vi "Load Firmware Data.vi"(8 "Error In":errorcluster, 9 "Firmware Index":i32, 10 "Device Index":i32, 11 "Family Index":i32) -> (0 "Error Out":errorcluster, 2 "Firmware Interface":T1, 3 "Firmware Description":string)   [LabVIEW 2011, in "LVH-LINX.lvlib"]
doc: "Load specified firmware readme."
uses:
  LVH-LINX.lvlib
  Device/Type Defs/Firmware Interface.ctl
  Type Defs/All Firmware Data FGV States.ctl
panel:
  in  "Device Family":u16(ring) items=["National Instruments", "Digilent", "Arduino"]
  in  "Device Type":u16(ring) items=["chipKIT Uno32", "chipKIT uC32", "chipKIT Max32", "chipKIT DP32"]
  in  "Firmware Version":u16(ring) items=["LINX -  Serial / USB", "LINX -  Serial / USB [Debug] "]
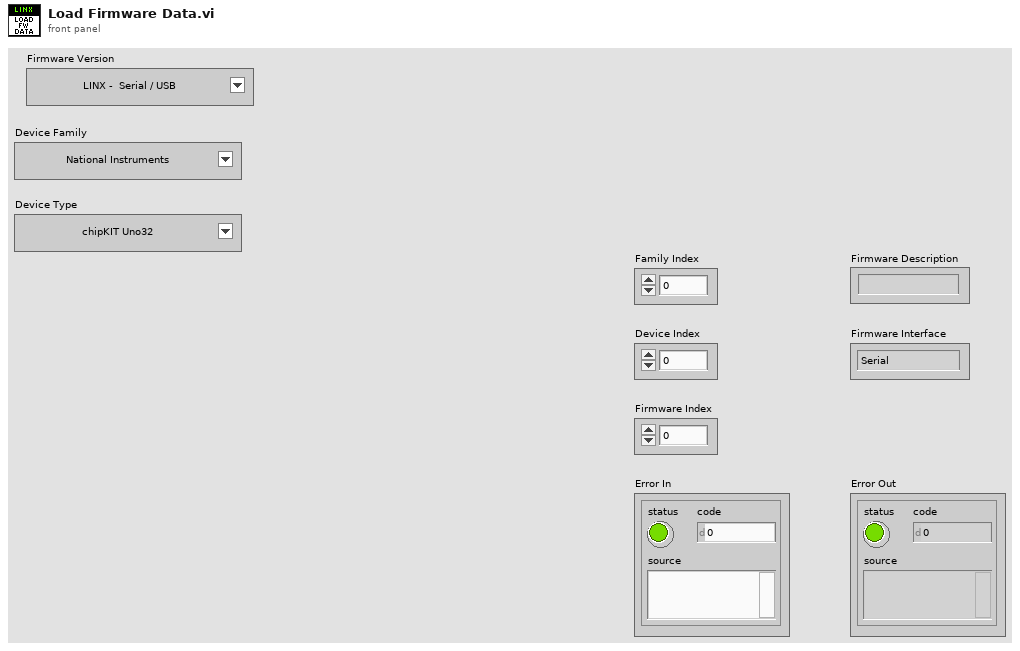
[diagram p1: front panel]
types:
  T1 = typedef "LVH-LINX.lvlib/Firmware Interface.ctl" = enum32{"Serial ", "Ethernet", "WIFI"}
  T2 = typedef "LVH-LINX.lvlib/All Firmware Data FGV States.ctl" = enum16{"Set", "Get"}
  T3 = typedef "LVH-LINX.lvlib/Device Firmware.ctl" = cluster{"Firmware Name":string, "Firmware Path":path, "Description":string, "LINX Interface":string, "Flash Util Working Dir":path, "Flash Util Name":string, "Flash Util Args":string, "Flash Timeout (ms)":i32}
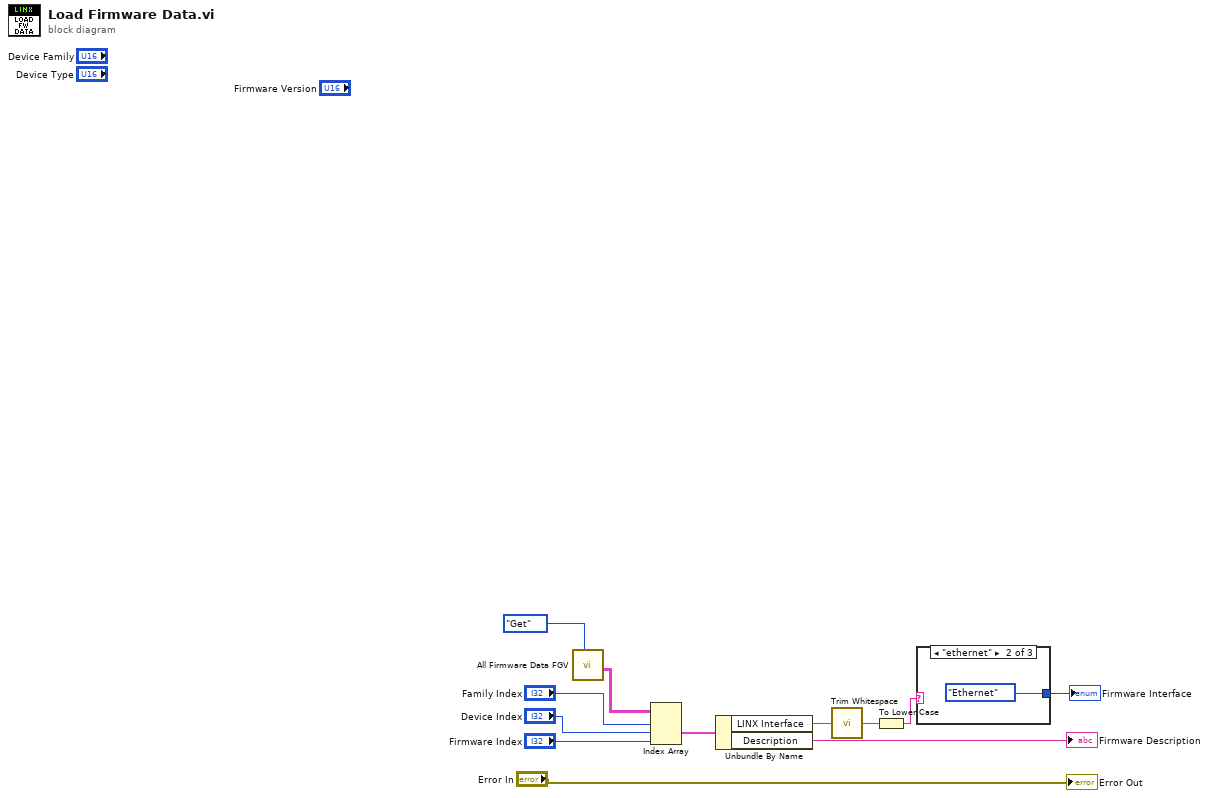
[diagram p0: block diagram]
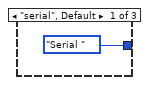
[diagram p2: hidden frame]
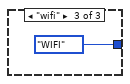
[diagram p3: hidden frame]
diagram:
  n1 = call "All Firmware Data FGV.vi"("All Firmware Data FGV States"=All_Firmware_Data_FGV_States."Get") -> ("Firmwares"=w11:T3[][][])  [unwired: 7 in, 3 out]
  n2 = Index Array(array=w11, index (dim 0)="Family Index", index (dim 1)="Device Index", index (dim 2)="Firmware Index") -> (element=w10:T3)
  n3 = Unbundle By Name(w10) -> ("LINX Interface"=w2:string, "Description"=→"Firmware Description":string)
  n4 = call <vilib>:"Trim Whitespace.vi"("string"=w2) -> ("trimmed string"=w5:string)  [unwired: 1 in]
  n5 = To Lower Case(string=w5) -> (all lower case string=w4:string)
  n6 = case shown="\"ethernet\"" w4 {
    tunnel: [Firmware_Interface."Serial " ("Firmware Interface") Firmware_Interface."Ethernet" ("Firmware Interface") Firmware_Interface."WIFI" ("Firmware Interface")] -> w3
    frame "serial", Default {
    }
    frame "ethernet" {
    }
    frame "wifi" {
    }
  }
  "Firmware Interface" <- w3
  "Error Out" <- "Error In"
